vi "readFilterData.vi"() -> ()   [LabVIEW 2026]
uses:
  <vilib>/Utility/miscctls.llb/LVRectTypeDef.ctl
  <vilib>/Utility/miscctls.llb/LVPointTypeDef.ctl
  <userlib>/Sensor.ctl
  <vilib>/Instr/_visa.llb/VISA Configure Serial Port (Instr).vi
panel:
  out "Result 2":dbl
  out "SyncStop 2":bool
  out "Freq Show 2":enum16{"1", "10", "100", "1000"}(ring)
  out "Result":dbl
  in  "UvodniStranka":bool
  in  "ExitApp":bool
  in  "error in (no error)":errorcluster
  in  "Tab Control":T1(tab)
  in  "Playground":bool
  in  "UlohaACC":bool
  in  "UlohaEDA":bool
  in  "UlohaEEG":bool
  in  "UlohaEMG":bool
  in  "UlohaEKG":bool
  out "GraphEKG":waveform(dbl)(graph)
  out "ChartEKG":dbl(graph)
  in  "Vstupní COM port 2":refnum<visa-resource-name>
  in  "Vzorkovací frekvence 2":enum16{"1", "10", "100", "1000"}(ring)
  out "Waveform Graph":waveform(dbl)(graph)
  in  "Cluster":T2
  in  "SendToFilter":bool
  out "Waveform Chart":dbl(graph)
  out "Waveform":waveform(dbl)(graph)
  out "SyncStop":bool
  in  "Vstupní COM port":refnum<visa-resource-name>
  in  "Vzorkovací frekvence (Hz)":enum16{"1", "10", "100", "1000"}(ring)
  in  "Druh signálu":T3
  in  "StartMeasure":bool
  in  "StopMeasure":bool
  in  "Radio Buttons":T4(radio)
  # "Aplikace pro mìøení na platformì PLUX BITalino"
  # "EKG"
  # "EEG"
  # "EDA"
  # "ACC"
  # "EMG"
  # "A1"
  # "A2"
  # "A3"
  # "A4"
  # "A5"
  # "A6"
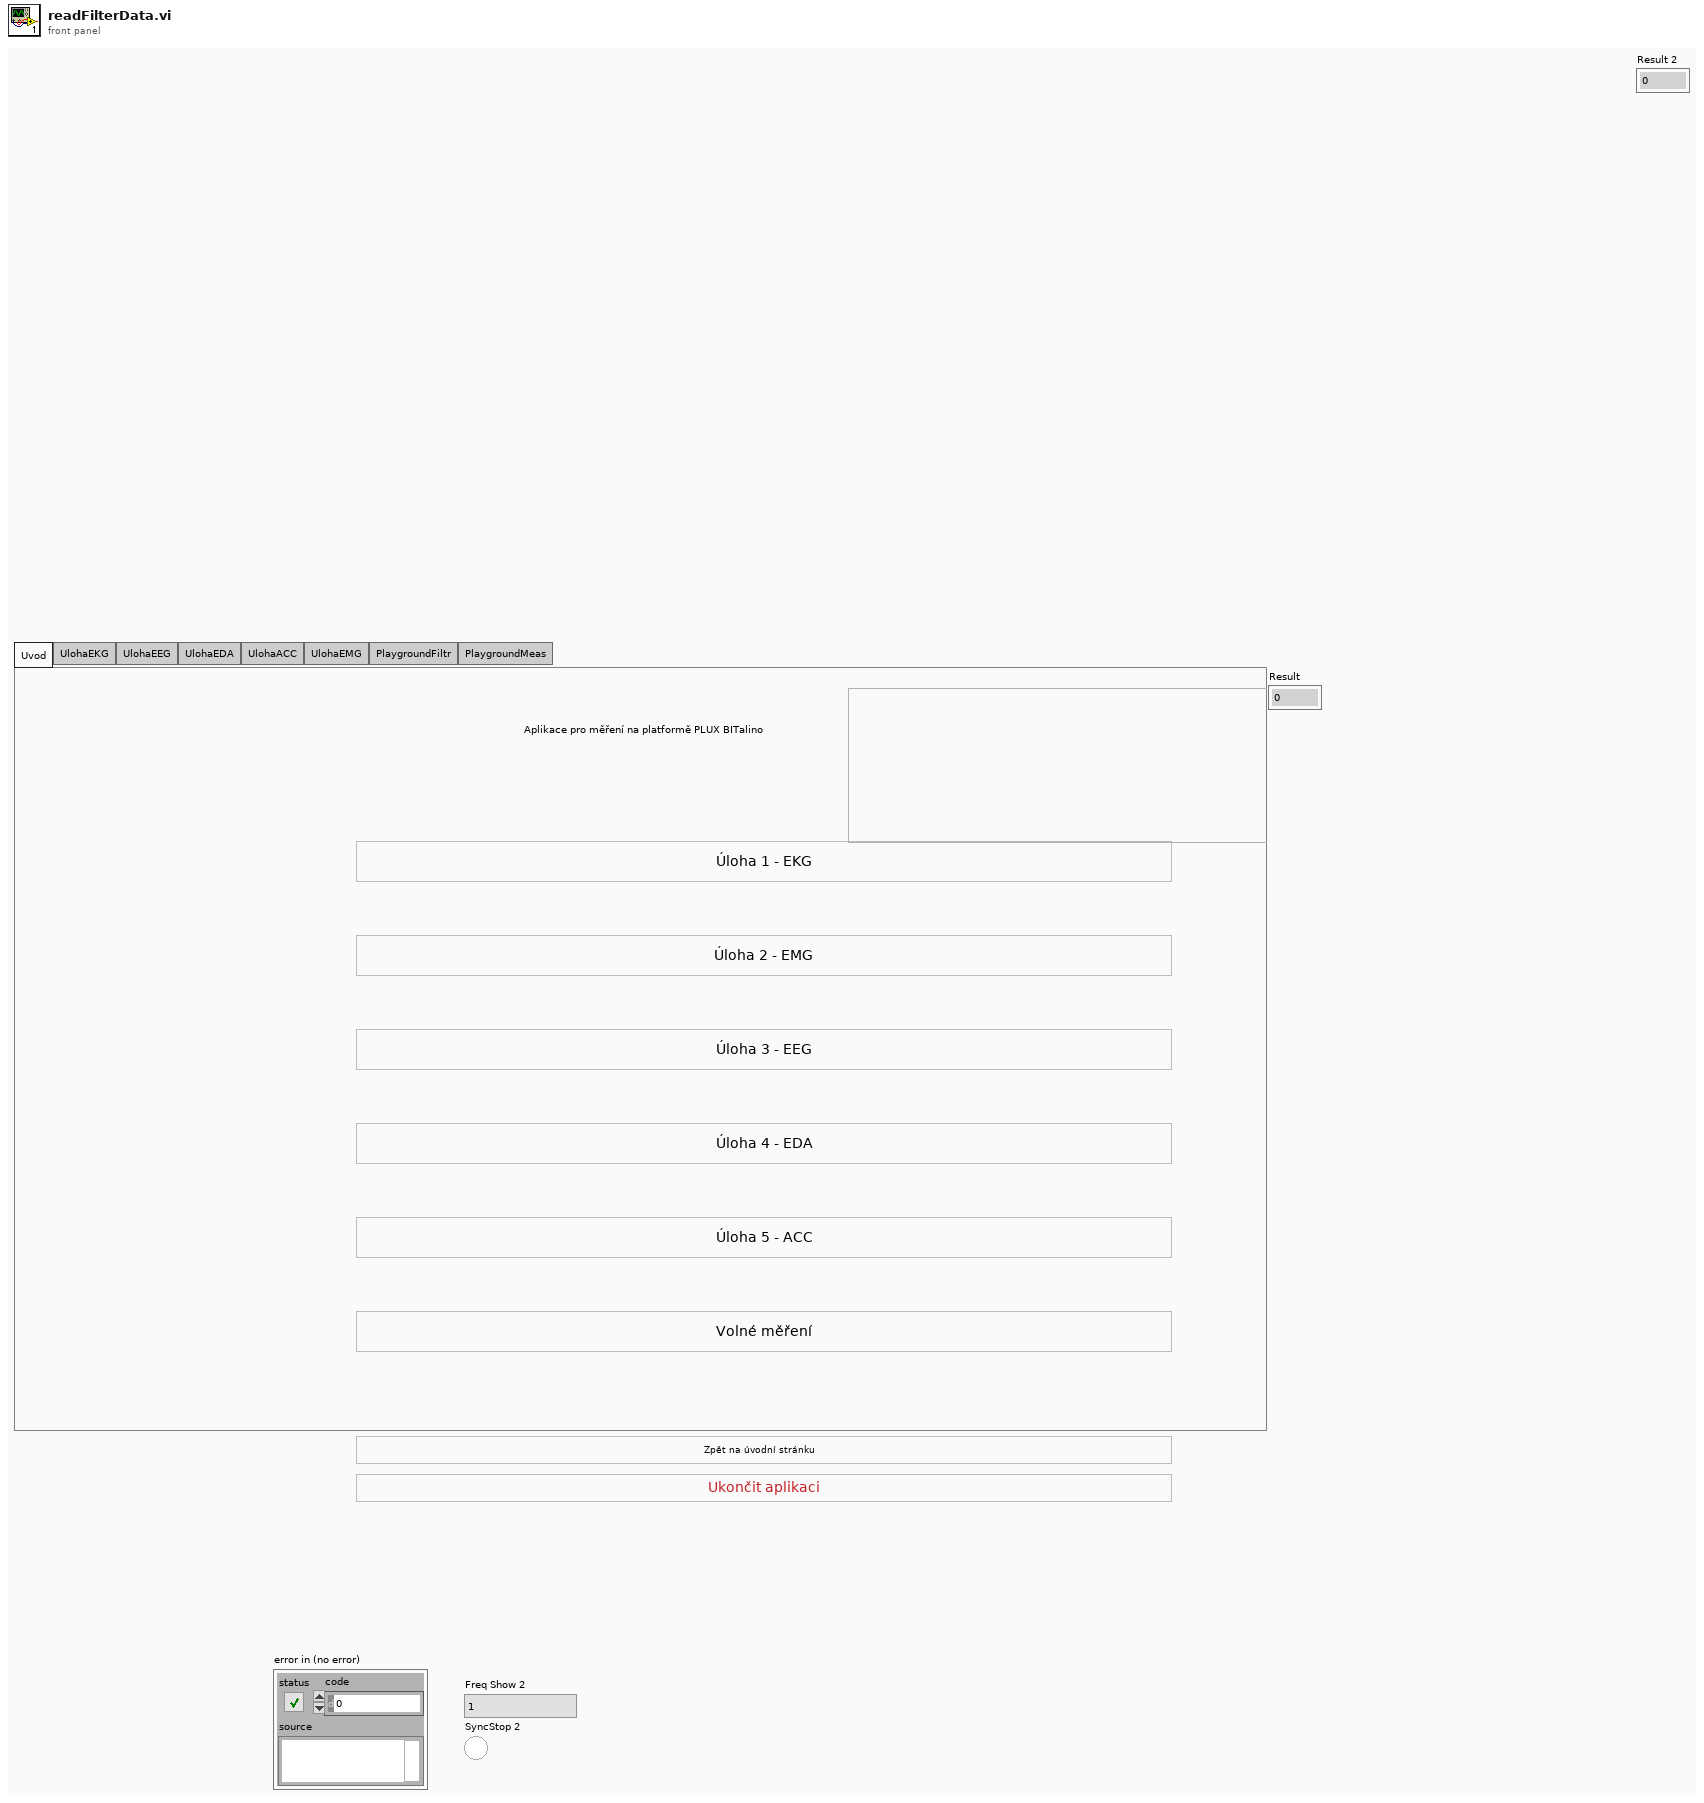
[diagram p1: front panel]
types:
  T1 = enum32{"Uvod", "UlohaEKG", "UlohaEEG", "UlohaEDA", "UlohaACC", "UlohaEMG", "PlaygroundFiltr", "PlaygroundMeas"}
  T2 = cluster{"Horní mezní frekvence":dbl, "Dolní mezní frekvence":dbl, "Filtr":bool, "OdstranitFiltr":bool, "filter type":enum32{"Lowpass", "Highpass", "Bandpass", "Bandstop"}}
  T3 = cluster{"Signál na kanálu A1":enum16{"EMG", "ECG", "EEG", "EDA", "ACC"}, "Signál na kanálu A2":enum16{"EMG", "ECG", "EEG", "EDA", "ACC"}, "Signál na kanálu A3":enum16{"EMG", "ECG", "EEG", "EDA", "ACC"}, "Signál na kanálu A4":enum16{"EMG", "ECG", "EEG", "EDA", "ACC"}, "Signál na kanálu A5":enum16{"EMG", "ECG", "EEG", "EDA", "ACC"}, "Signál na kanálu A6":enum16{"EMG", "ECG", "EEG", "EDA", "ACC"}}
  T4 = enum32{"Item 0", "Item 1", "Item 2", "Item 3", "Item 4", "Item 5"}
  T5 = enum16{"Wait", "Exit", "Measure", "Intro", "UlohaEKG", "UlohaEMG", "PlaygroundMeas", "UlohaEEG", "UlohaEDA", "UlohaACC", "PlaygroundFiltr"}
  T6 = enum16{"Always On", "Always Off", "Off While Running"}
  T7 = enum32{"Uvod", "UlohaEKG", "UlohaEEG", "UlohaEDA", "UlohaACC", "UlohaEMG", "PlaygroundFiltr"}
  T8 = typedef "LVPointTypeDef.ctl" = cluster{"Horizontal":i16, "Vertical":i16}
  T9 = typedef "LVRectTypeDef.ctl" = cluster{"Left":i16, "Top":i16, "Right":i16, "Bottom":i16}
  T10 = enum16{"Wait", "Exit", "Measure", "Intro", "UlohaEKG", "UlohaEMG", "PlaygroundMeas", "UlohaEEG", "UlohaEDA", "UlohaACC"}
  T11 = enum16{"Wait", "Exit", "Measure", "Intro", "UlohaEKG", "UlohaEMG", "PlaygroundMeas"}
  T12 = enum16{"Wait", "Exit", "Measure", "Intro", "UlohaEKG", "UlohaEMG"}
  T13 = enum8{"Enabled", "Disabled", "Disabled and Grayed Out"}
  T14 = typedef "Sensor.ctl" = enum16{"EMG", "ECG", "EEG", "EDA", "ACC", "LUX"}
  T15 = cluster{"Sensor 1":T14, "Sensor 2":T14, "Sensor 3":T14, "Sensor 4":T14, "Sensor 5":T14, "Sensor 6":T14}
  T16 = cluster{"Result":dbl, "Result":dbl, "Result":dbl, "Result":dbl, "Result":dbl, "Result":dbl}
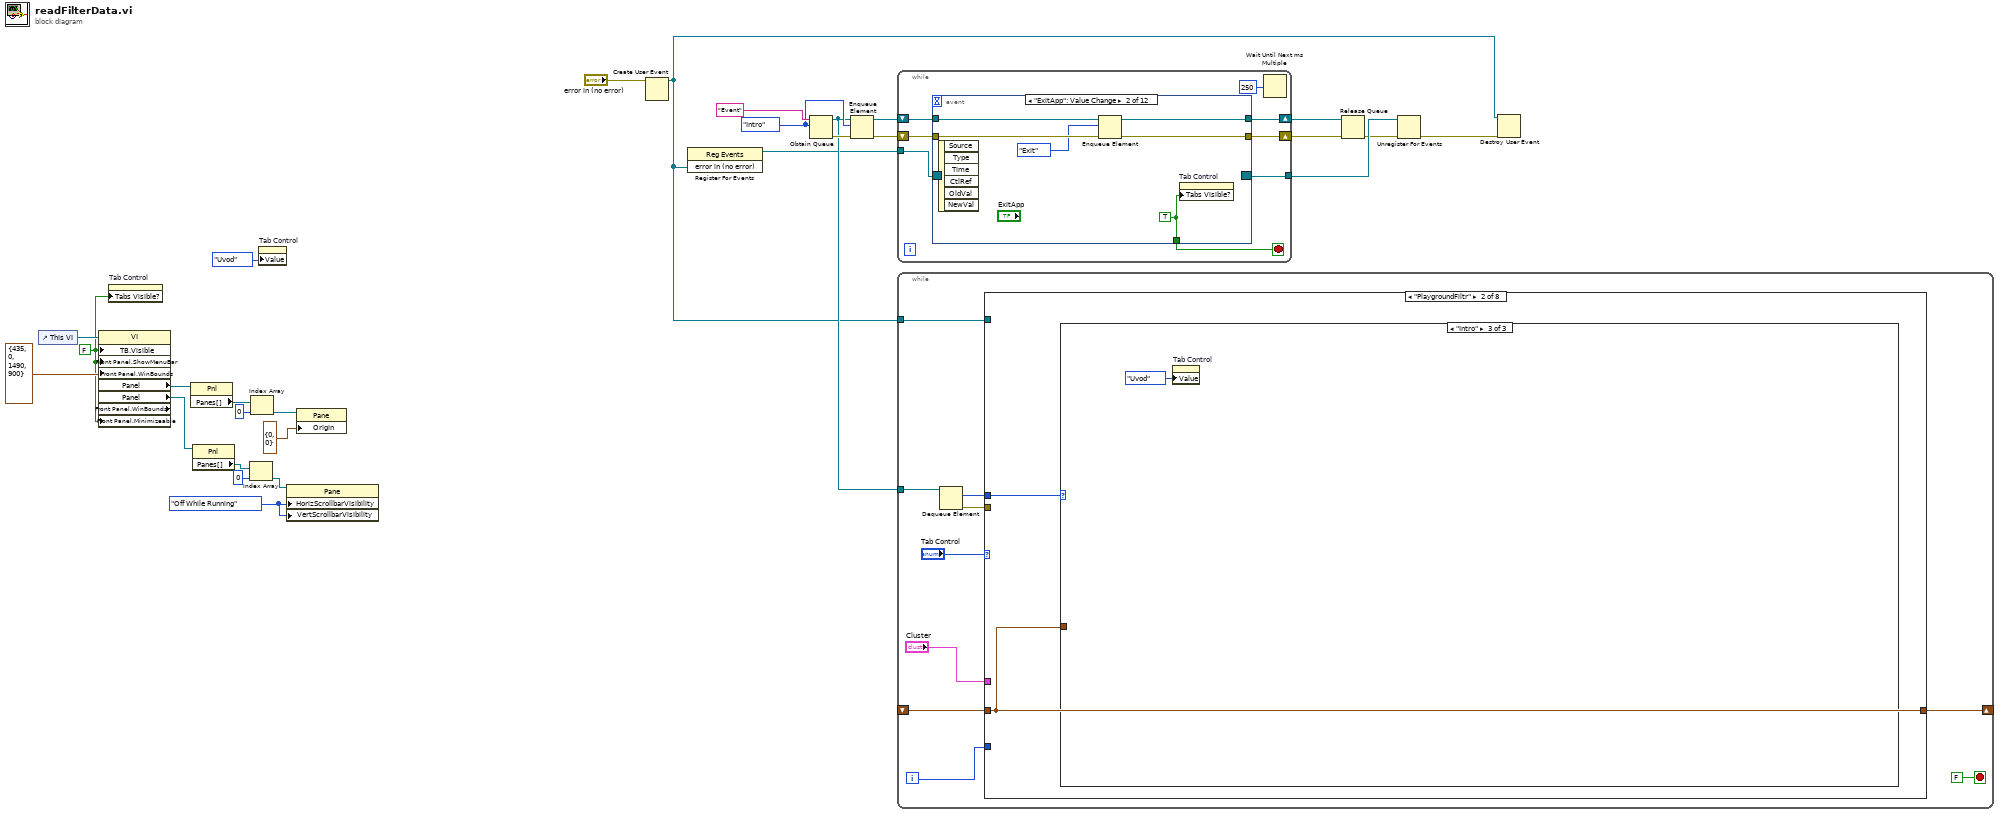
[diagram p0: block diagram]
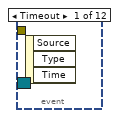
[diagram p2: hidden frame]
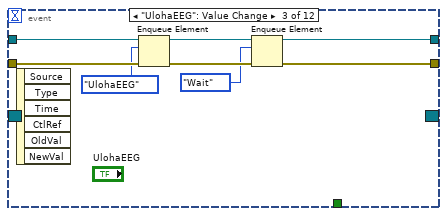
[diagram p3: hidden frame]
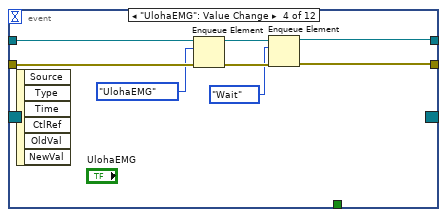
[diagram p4: hidden frame]
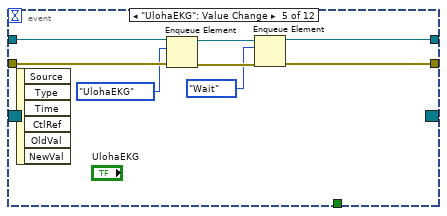
[diagram p5: hidden frame]
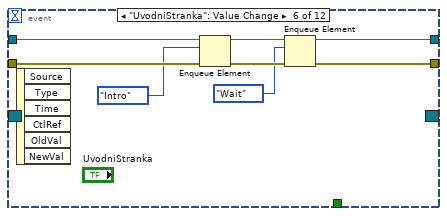
[diagram p6: hidden frame]
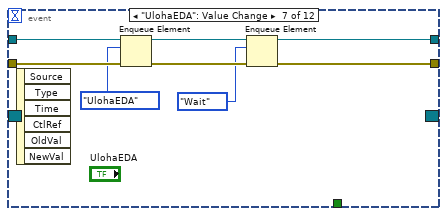
[diagram p7: hidden frame]
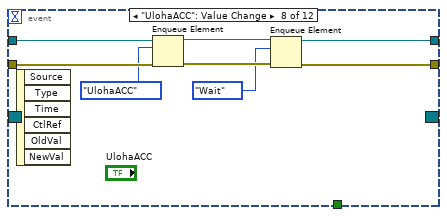
[diagram p8: hidden frame]
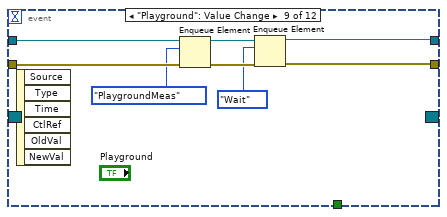
[diagram p9: hidden frame]
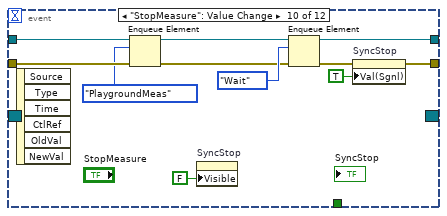
[diagram p10: hidden frame]
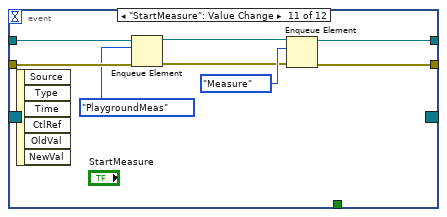
[diagram p11: hidden frame]
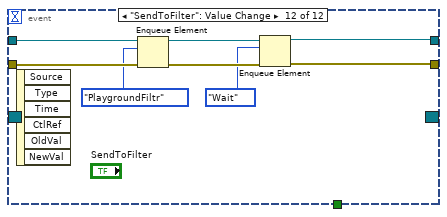
[diagram p12: hidden frame]
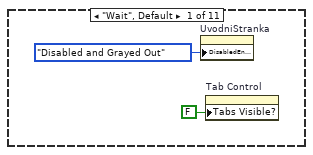
[diagram p14: hidden frame]
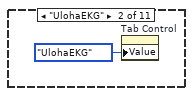
[diagram p15: hidden frame]
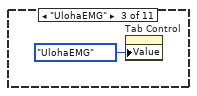
[diagram p16: hidden frame]
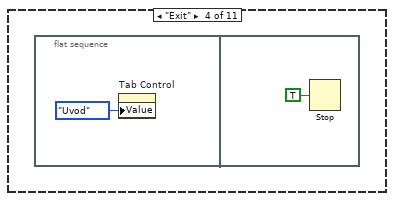
[diagram p17: hidden frame]
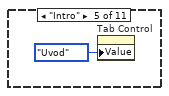
[diagram p18: hidden frame]
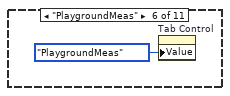
[diagram p19: hidden frame]
diagram:
  w10 = T5."Intro"
  w16 = T6."Off While Running" ("Horizontal Scrollbar Visibility")
  w15 = FALSE ("Front Panel Window:Closeable")
  n1 = control-ref of="This VI"() -> (w28:refnum<vi>)
  n2 = property class="VI" props=["TB.Visible", "Front Panel.ShowMenuBar", "Front Panel.WinBounds", "Panel", "Panel", "Front Panel.WinBounds", "Front Panel.Minimizeable"](reference=w28, "TB.Visible"=w15, "Front Panel.ShowMenuBar"=w15, "Front Panel.WinBounds"=T9 {"Left"=435, "Top"=0, "Right"=1490, "Bottom"=900} ("Front Panel Window:Window Bounds"), "Front Panel.Minimizeable"=w15) -> ("Panel"=w26:refnum<vi>, "Panel"=w20:refnum<vi>)  [unwired: 1 in, 3 out]
  n3 = property on="Tab Control" class="TabCtl (strict)"("Tabs Visible?"=w15) -> ()  [unwired: 2 in, 2 out]
  n4 = property class="Pnl"(reference=w26) -> ("Panes[]"=w25:refnum<vi>[])  [unwired: 1 in, 2 out]
  n5 = property class="Pnl"(reference=w20) -> ("Panes[]"=w19:refnum<vi>[])  [unwired: 1 in, 2 out]
  n6 = Index Array(array=w19, index=0) -> (element=w17:refnum<vi>)
  n7 = Index Array(array=w25, index=0) -> (element=w23:refnum<vi>)
  n8 = property on="Tab Control" class="TabCtl (strict)"("Value"=T7."Uvod" ("Tab Control")) -> ()  [unwired: 2 in, 2 out]
  n9 = property class="Pane"(reference=w17, "HorizScrollbarVisibility"=w16, "VertScrollbarVisibility"=w16) -> ()  [unwired: 1 in, 2 out]
  n10 = property class="Pane"(reference=w23, "Origin"=T8 {"Horizontal"=0, "Vertical"=0}) -> ()  [unwired: 1 in, 2 out]
  n11 = Create User Event(user event datatype="error in (no error)") -> (user event=w2:refnum<user-event>)  [unwired: 1 in, 1 out]
  n12 = register-events(w2) -> (reference out=w1:refnum<event-registration>)  [unwired: 2 in, 1 out]
  n13 = Obtain Queue(name (unnamed)="Event", element data type=w10) -> (queue out=w9:refnum<queue>, error out=w13:errorcluster)  [unwired: 3 in, 1 out]
  n14 = Enqueue Element(queue=w9, element=w10, error in (no error)=w13) -> (queue out=w12:refnum<queue>, error out=w11:errorcluster)  [unwired: 1 in, 1 out]
  n15 = while {
    shift-right: [w34] -> w7
    shift-left: w11 -> [w33]
    shift-right: [w35] -> w8
    shift-left: w12 -> [w36]
    tunnel: [w30] -> w5
    tunnel: w1 -> [w29]
    stop <- w32 stop-if-true
    n16 = event shown="[1] \"ExitApp\": Value Change" {
      selector: w29 -> [_ _ _ _ _ _ _ _ _ _ _ _]
      dyn-events: [_ _ _ _ _ _ _ _ _ _ _ _] -> w30
      timeout: _ -> [_ _ _ _ _ _ _ _ _ _ _ _]
      tunnel: w36 -> [_ w42 w50 w58 w66 w74 w82 w90 w98 w103 w114 w125]
      tunnel: w33 -> [_ w41 w49 w57 w65 w73 w81 w89 w97 w101 w112 w124]
      tunnel: [_ w40 w46 w54 w62 w69 w79 w87 w92 w108 w117 w121] -> w35
      tunnel: [_ w39 w44 w53 w60 w68 w78 w85 w94 w105 w116 w119] -> w34
      tunnel: [_ w37 _ _ _ _ _ _ _ _ _ _] -> w32
      event Timeout {
        n17 = event-data() -> ()  [unwired: 1 in, 3 out]
      }
      event "ExitApp": Value Change {
        w37 = TRUE
        n18 = event-data() -> ()  [unwired: 1 in, 6 out]
        n19 = Enqueue Element(queue=w42, element=enum16{"Wait", "Exit", "Measure"}."Exit", error in (no error)=w41) -> (queue out=w40:refnum<queue>, error out=w39:errorcluster)  [unwired: 1 in, 1 out]
        n20 = property on="Tab Control" class="TabCtl (strict)"("Tabs Visible?"=w37) -> ()  [unwired: 2 in, 2 out]
      }
      event "UlohaEEG": Value Change {
        n21 = event-data() -> ()  [unwired: 1 in, 6 out]
        n22 = Enqueue Element(queue=w50, element=T10."UlohaEEG", error in (no error)=w49) -> (queue out=w47:refnum<queue>, error out=w45:errorcluster)  [unwired: 1 in, 1 out]
        n23 = Enqueue Element(queue=w47, element=T10."Wait", error in (no error)=w45) -> (queue out=w46:refnum<queue>, error out=w44:errorcluster)  [unwired: 1 in, 1 out]
      }
      event "UlohaEMG": Value Change {
        n24 = event-data() -> ()  [unwired: 1 in, 6 out]
        n25 = Enqueue Element(queue=w58, element=T11."UlohaEMG", error in (no error)=w57) -> (queue out=w55:refnum<queue>, error out=w52:errorcluster)  [unwired: 1 in, 1 out]
        n26 = Enqueue Element(queue=w55, element=T11."Wait", error in (no error)=w52) -> (queue out=w54:refnum<queue>, error out=w53:errorcluster)  [unwired: 1 in, 1 out]
      }
      event "UlohaEKG": Value Change {
        n27 = event-data() -> ()  [unwired: 1 in, 6 out]
        n28 = Enqueue Element(queue=w66, element=T12."UlohaEKG", error in (no error)=w65) -> (queue out=w63:refnum<queue>, error out=w61:errorcluster)  [unwired: 1 in, 1 out]
        n29 = Enqueue Element(queue=w63, element=T12."Wait", error in (no error)=w61) -> (queue out=w62:refnum<queue>, error out=w60:errorcluster)  [unwired: 1 in, 1 out]
      }
      event "UvodniStranka": Value Change {
        n30 = event-data() -> ()  [unwired: 1 in, 6 out]
        n31 = Enqueue Element(queue=w74, element=T12."Intro", error in (no error)=w73) -> (queue out=w71:refnum<queue>, error out=w70:errorcluster)  [unwired: 1 in, 1 out]
        n32 = Enqueue Element(queue=w71, element=T12."Wait", error in (no error)=w70) -> (queue out=w69:refnum<queue>, error out=w68:errorcluster)  [unwired: 1 in, 1 out]
      }
      event "UlohaEDA": Value Change {
        n33 = event-data() -> ()  [unwired: 1 in, 6 out]
        n34 = Enqueue Element(queue=w82, element=T10."UlohaEDA", error in (no error)=w81) -> (queue out=w80:refnum<queue>, error out=w77:errorcluster)  [unwired: 1 in, 1 out]
        n35 = Enqueue Element(queue=w80, element=T10."Wait", error in (no error)=w77) -> (queue out=w79:refnum<queue>, error out=w78:errorcluster)  [unwired: 1 in, 1 out]
      }
      event "UlohaACC": Value Change {
        n36 = event-data() -> ()  [unwired: 1 in, 6 out]
        n37 = Enqueue Element(queue=w90, element=T10."UlohaACC", error in (no error)=w89) -> (queue out=w88:refnum<queue>, error out=w86:errorcluster)  [unwired: 1 in, 1 out]
        n38 = Enqueue Element(queue=w88, element=T10."Wait", error in (no error)=w86) -> (queue out=w87:refnum<queue>, error out=w85:errorcluster)  [unwired: 1 in, 1 out]
      }
      event "Playground": Value Change {
        n39 = event-data() -> ()  [unwired: 1 in, 6 out]
        n40 = Enqueue Element(queue=w98, element=T11."PlaygroundMeas", error in (no error)=w97) -> (queue out=w93:refnum<queue>, error out=w95:errorcluster)  [unwired: 1 in, 1 out]
        n41 = Enqueue Element(queue=w93, element=T11."Wait", error in (no error)=w95) -> (queue out=w92:refnum<queue>, error out=w94:errorcluster)  [unwired: 1 in, 1 out]
      }
      event "StopMeasure": Value Change {
        n42 = event-data() -> ()  [unwired: 1 in, 6 out]
        n43 = Enqueue Element(queue=w103, element=T11."PlaygroundMeas", error in (no error)=w101) -> (queue out=w102:refnum<queue>, error out=w100:errorcluster)  [unwired: 1 in, 1 out]
        n44 = property on="SyncStop" class="Bool (strict)"("Visible"=FALSE) -> ()  [unwired: 2 in, 2 out]
        n45 = Enqueue Element(queue=w102, element=enum16{"Wait", "Exit", "Measure"}."Wait", error in (no error)=w100) -> (queue out=w108:refnum<queue>, error out=w106:errorcluster)  [unwired: 1 in, 1 out]
        n46 = property on="SyncStop" class="Bool (strict)"(error in=w106, "Val(Sgnl)"=TRUE ("Value (Signaling)")) -> (error out=w105:errorcluster)  [unwired: 1 in, 1 out]
      }
      event "StartMeasure": Value Change {
        n47 = event-data() -> ()  [unwired: 1 in, 6 out]
        n48 = Enqueue Element(queue=w114, element=T11."PlaygroundMeas", error in (no error)=w112) -> (queue out=w113:refnum<queue>, error out=w111:errorcluster)  [unwired: 1 in, 1 out]
        n49 = Enqueue Element(queue=w113, element=enum16{"Wait", "Exit", "Measure"}."Measure", error in (no error)=w111) -> (queue out=w117:refnum<queue>, error out=w116:errorcluster)  [unwired: 1 in, 1 out]
      }
      event "SendToFilter": Value Change {
        n50 = event-data() -> ()  [unwired: 1 in, 6 out]
        n51 = Enqueue Element(queue=w125, element=T5."PlaygroundFiltr", error in (no error)=w124) -> (queue out=w122:refnum<queue>, error out=w120:errorcluster)  [unwired: 1 in, 1 out]
        n52 = Enqueue Element(queue=w122, element=T5."Wait", error in (no error)=w120) -> (queue out=w121:refnum<queue>, error out=w119:errorcluster)  [unwired: 1 in, 1 out]
      }
    }
    n53 = Wait Until Next ms Multiple(millisecond multiple=u32 250) -> ()  [unwired: 1 out]
  }
  n54 = while {
    shift-right: [w135] -> _
    shift-left: _ -> [w134]
    tunnel: w9 -> [w129]
    tunnel: w2 -> [w128]
    i -> [w132]
    stop <- FALSE stop-if-true
    n55 = Dequeue Element(queue=w129) -> (element=w130:T5, error out=w127:errorcluster)  [unwired: 2 in, 2 out]
    n56 = case shown="\"PlaygroundFiltr\"" "Tab Control" {
      tunnel: [w137 w149 w158 w223 w229 w235 w241 w247] -> w135
      tunnel: w134 -> [w137 w149 w158 w223 w229 w235 w241 w246]
      tunnel: "Cluster" -> [_ _ _ _ _ _ _ _]
      tunnel: w132 -> [_ _ _ _ _ _ _ _]
      tunnel: w130 -> [w136 w150 w157 w222 w228 w234 w240 w250]
      tunnel: w128 -> [_ _ w156 _ _ _ _ w249]
      tunnel: w127 -> [_ _ _ _ _ _ _ w248]
      frame "Uvod", Default {
        n57 = case shown="\"PlaygroundFiltr\"" w136 {
          frame "Wait", Default {
            n58 = property on="UvodniStranka" class="Bool"("DisabledEnum"=T13."Disabled and Grayed Out" ("Disabled")) -> ()  [unwired: 2 in, 2 out]
            n59 = property on="Tab Control" class="TabCtl (strict)"("Tabs Visible?"=FALSE) -> ()  [unwired: 2 in, 2 out]
          }
          frame "UlohaEKG" {
            n60 = property on="Tab Control" class="TabCtl (strict)"("Value"=T1."UlohaEKG" ("Tab Control")) -> ()  [unwired: 2 in, 2 out]
          }
          frame "UlohaEMG" {
            n61 = property on="Tab Control" class="TabCtl (strict)"("Value"=T1."UlohaEMG" ("Tab Control")) -> ()  [unwired: 2 in, 2 out]
          }
          frame "Exit" {
            n62 = flat-sequence {
              frame #0 {
                n63 = property on="Tab Control" class="TabCtl (strict)"("Value"=T1."Uvod" ("Tab Control")) -> ()  [unwired: 2 in, 2 out]
              }
              frame #1 {
                n64 = Stop(stop? (T)=TRUE) -> ()
              }
            }
          }
          frame "Intro" {
            n65 = property on="Tab Control" class="TabCtl (strict)"("Value"=T1."Uvod" ("Tab Control")) -> ()  [unwired: 2 in, 2 out]
          }
          frame "PlaygroundMeas" {
            n66 = property on="Tab Control" class="TabCtl (strict)"("Value"=T1."PlaygroundMeas" ("Tab Control")) -> ()  [unwired: 2 in, 2 out]
          }
          frame "Measure" {
          }
          frame "UlohaEEG" {
            n67 = property on="Tab Control" class="TabCtl (strict)"("Value"=T1."UlohaEEG" ("Tab Control")) -> ()  [unwired: 2 in, 2 out]
          }
          frame "UlohaEDA" {
            n68 = property on="Tab Control" class="TabCtl (strict)"("Value"=T1."UlohaEDA" ("Tab Control")) -> ()  [unwired: 2 in, 2 out]
          }
          frame "UlohaACC" {
            n69 = property on="Tab Control" class="TabCtl (strict)"("Value"=T1."UlohaACC" ("Tab Control")) -> ()  [unwired: 2 in, 2 out]
          }
          frame "PlaygroundFiltr" {
          }
        }
      }
      frame "PlaygroundFiltr" {
        n70 = case shown="\"Intro\"" w150 {
          tunnel: w149 -> [w151 _ _]
          frame "Wait", Default {
            n71 = property on="UvodniStranka" class="Bool"("DisabledEnum"=T13."Enabled" ("Disabled")) -> ()  [unwired: 2 in, 2 out]
            "Waveform Graph" <- w151
          }
          frame "Exit" {
            n72 = flat-sequence {
              frame #0 {
                n73 = property on="Tab Control" class="TabCtl (strict)"("Value"=T1."Uvod" ("Tab Control")) -> ()  [unwired: 2 in, 2 out]
              }
              frame #1 {
                n74 = Stop(stop? (T)=TRUE) -> ()
              }
            }
          }
          frame "Intro" {
            n75 = property on="Tab Control" class="TabCtl (strict)"("Value"=T1."Uvod" ("Tab Control")) -> ()  [unwired: 2 in, 2 out]
          }
        }
      }
      frame "UlohaEKG" {
        n76 = case shown="\"Intro\"" w157 {
          tunnel: w156 -> [_ _ w166 _ _ _]
          frame "Wait", Default {
            n77 = property on="UvodniStranka" class="Bool"("DisabledEnum"=T13."Enabled" ("Disabled")) -> ()  [unwired: 2 in, 2 out]
          }
          frame "Exit" {
            n78 = flat-sequence {
              frame #0 {
                n79 = property on="Tab Control" class="TabCtl (strict)"("Value"=T1."Uvod" ("Tab Control")) -> ()  [unwired: 2 in, 2 out]
              }
              frame #1 {
                n80 = Stop(stop? (T)=TRUE) -> ()
              }
            }
          }
          frame "Measure" {
            w169 = "Signal" ("name (unnamed)")
            n81 = call-poly "VISA Configure Serial Port"("VISA resource name"="Vstupní COM port 2", "timeout (10sec)"=u32 2000, "baud rate (9600)"=u32 115200) -> ("VISA resource name out"=w186:refnum<visa-resource-name>, "error out"=w185:errorcluster)  [unwired: 11 in]
            n82 = call "InitBITalino.vi"("Battery \nThreshold (%)"=u8 5 ("Battery \nThreshold (%)"), "MODE"=FALSE, "error in (no error)"=w185, "Sample Rate"="Vzorkovací frekvence 2", "BITalino"=w186) -> ("error out"=w181:errorcluster, "VISA out"=w182:refnum<visa-resource-name>)  [unwired: 4 in, 1 out]
            n83 = Obtain Queue(name (unnamed)=w169, element data type=w169, error in (no error)=w181) -> (queue out=w165:refnum<queue>, error out=w180:errorcluster)  [unwired: 2 in, 1 out]
            n84 = while {
              tunnel: w165 -> [w194]
              tunnel: [w190] -> w164 mode=indexing
              stop <- w191 stop-if-true
              n85 = Dequeue Element(queue=w194) -> (element=w193:string, error out=w192:errorcluster)  [unwired: 2 in, 2 out]
              n86 = case shown="No Error" w192 {
                tunnel: w193 -> [w203 _]
                tunnel: [FALSE TRUE] -> w191
                tunnel: [w197 w204] -> w190
                frame No Error {
                  n87 = call "Packet Read.vi"("Packets"=w203) -> ("Analog Channels"=w202:cluster{u16, u16, u16, u16, u16, u16})  [unwired: 7 in, 3 out]
                  n88 = call "Conversion.vi"("Sensor Type"=T15 {"Sensor 1"=enum."ECG", "Sensor 2"=enum."ECG", "Sensor 3"=enum."ECG", "Sensor 4"=enum."ECG", "Sensor 5"=enum."ECG", "Sensor 6"=enum."ECG"}, "Analog Channels"=w202) -> ("output cluster"=w200:T16)  [unwired: 8 in, 1 out]
                  n89 = Cluster To Array(cluster=w200) -> (array=w199:dbl[])
                  n90 = Unbundle(w200) -> ("Result"=w197:dbl)  [unwired: 5 out]
                  "Result 2" <- w197
                  n91 = Index Array(array=w199, index=2) -> (element=→"ChartEKG":dbl)
                }
                frame Error {
                  n92 = local read "Result 2"() -> (w204:dbl)
                }
              }
            }
            n93 = while {
              shift-right: [w214] -> w178
              shift-left: w182 -> [w220]
              shift-right: [w209] -> w179
              shift-left: w180 -> [w219]
              shift-right: [w210] -> w173
              shift-left: w165 -> [w213]
              stop <- w208 stop-if-true
              n94 = VISA Write(VISA resource name=w220, write buffer="0x03", error in (no error)=w219) -> (VISA resource name out=w217:refnum<visa-resource-name>, error out=w216:errorcluster)  [unwired: 1 out]
              n95 = VISA Read(VISA resource name=w217, byte count=u32 8, error in (no error)=w216) -> (VISA resource name out=w214:refnum<visa-resource-name>, read buffer=w212:string, error out=w211:errorcluster)  [unwired: 1 out]
              n96 = Enqueue Element(queue=w213, element=w212, error in (no error)=w211) -> (queue out=w210:refnum<queue>, error out=w209:errorcluster)  [unwired: 1 in, 1 out]
              n97 = local read "SyncStop 2"() -> (w206:bool)
              n98 = Unbundle By Name(w209) -> ("status"=w207:bool)
              n99 = Or(x=w207, y=w206) -> (x .or. y?=w208:bool)
            }
            n100 = call "Wait.vi"("error in (no error)"=w179) -> ("error out"=w175:errorcluster)  [unwired: 10 in]
            n101 = Build Array(u8 0) -> (w171:u8[])
            n102 = Byte Array To String(unsigned byte array=w171) -> (string=w170:string)
            n103 = VISA Write(VISA resource name=w178, write buffer=w170, error in (no error)=w175) -> (VISA resource name out=w177:refnum<visa-resource-name>, error out=w176:errorcluster)  [unwired: 1 out]
            n104 = VISA Close(VISA resource name=w177, error in (no error)=w176) -> (error out=w174:errorcluster)
            n105 = Bundle By Name("Y"=w164, "dt"=0.001) -> (→"GraphEKG":waveform(dbl))  [unwired: 1 in]
            n106 = Release Queue(queue=w173, error in (no error)=w174) -> (error out=w168:errorcluster)  [unwired: 1 in, 2 out]
            n107 = Generate User Event(user event=w166, event data cluster=w168) -> ()  [unwired: 2 in, 2 out]
            "Freq Show 2" <- "Vzorkovací frekvence 2"
          }
          frame "Intro" {
            n108 = property on="Tab Control" class="TabCtl (strict)"("Value"=T1."Uvod" ("Tab Control")) -> ()  [unwired: 2 in, 2 out]
          }
          frame "UlohaEKG" {
          }
          frame "UlohaEMG" {
          }
        }
      }
      frame "UlohaEEG" {
        n109 = case shown="\"Exit\"" w222 {
          frame "Wait", Default {
            n110 = property on="UvodniStranka" class="Bool"("DisabledEnum"=T13."Enabled" ("Disabled")) -> ()  [unwired: 2 in, 2 out]
          }
          frame "Exit" {
            n111 = flat-sequence {
              frame #0 {
                n112 = property on="Tab Control" class="TabCtl (strict)"("Value"=T1."Uvod" ("Tab Control")) -> ()  [unwired: 2 in, 2 out]
              }
              frame #1 {
                n113 = Stop(stop? (T)=TRUE) -> ()
              }
            }
          }
          frame "Measure" {
          }
          frame "Intro" {
            n114 = property on="Tab Control" class="TabCtl (strict)"("Value"=T1."Uvod" ("Tab Control")) -> ()  [unwired: 2 in, 2 out]
          }
          frame "UlohaEKG" {
          }
          frame "UlohaEMG" {
          }
          frame "PlaygroundMeas" {
          }
          frame "UlohaEEG" {
          }
          frame "UlohaEDA" {
          }
          frame "UlohaACC" {
          }
        }
      }
      frame "UlohaEDA" {
        n115 = case shown="\"Wait\", Default" w228 {
          frame "Wait", Default {
            n116 = property on="UvodniStranka" class="Bool"("DisabledEnum"=T13."Enabled" ("Disabled")) -> ()  [unwired: 2 in, 2 out]
          }
          frame "Exit" {
            n117 = flat-sequence {
              frame #0 {
                n118 = property on="Tab Control" class="TabCtl (strict)"("Value"=T1."Uvod" ("Tab Control")) -> ()  [unwired: 2 in, 2 out]
              }
              frame #1 {
                n119 = Stop(stop? (T)=TRUE) -> ()
              }
            }
          }
          frame "Measure" {
          }
          frame "Intro" {
            n120 = property on="Tab Control" class="TabCtl (strict)"("Value"=T1."Uvod" ("Tab Control")) -> ()  [unwired: 2 in, 2 out]
          }
          frame "UlohaEKG" {
          }
          frame "UlohaEMG" {
          }
          frame "PlaygroundMeas" {
          }
          frame "UlohaEEG" {
          }
          frame "UlohaEDA" {
          }
          frame "UlohaACC" {
          }
        }
      }
      frame "UlohaACC" {
        n121 = case shown="\"Wait\", Default" w234 {
          frame "Wait", Default {
            n122 = property on="UvodniStranka" class="Bool"("DisabledEnum"=T13."Enabled" ("Disabled")) -> ()  [unwired: 2 in, 2 out]
          }
          frame "Exit" {
            n123 = flat-sequence {
              frame #0 {
                n124 = property on="Tab Control" class="TabCtl (strict)"("Value"=T1."Uvod" ("Tab Control")) -> ()  [unwired: 2 in, 2 out]
              }
              frame #1 {
                n125 = Stop(stop? (T)=TRUE) -> ()
              }
            }
          }
          frame "Measure" {
          }
          frame "Intro" {
            n126 = property on="Tab Control" class="TabCtl (strict)"("Value"=T1."Uvod" ("Tab Control")) -> ()  [unwired: 2 in, 2 out]
          }
          frame "UlohaEKG" {
          }
          frame "UlohaEMG" {
          }
          frame "PlaygroundMeas" {
          }
          frame "UlohaEEG" {
          }
          frame "UlohaEDA" {
          }
          frame "UlohaACC" {
          }
        }
      }
      frame "UlohaEMG" {
        n127 = case shown="\"Intro\"" w240 {
          frame "Wait", Default {
            n128 = property on="UvodniStranka" class="Bool"("DisabledEnum"=T13."Enabled" ("Disabled")) -> ()  [unwired: 2 in, 2 out]
          }
          frame "Exit" {
            n129 = flat-sequence {
              frame #0 {
                n130 = property on="Tab Control" class="TabCtl (strict)"("Value"=T1."Uvod" ("Tab Control")) -> ()  [unwired: 2 in, 2 out]
              }
              frame #1 {
                n131 = Stop(stop? (T)=TRUE) -> ()
              }
            }
          }
          frame "Measure" {
          }
          frame "Intro" {
            n132 = property on="Tab Control" class="TabCtl (strict)"("Value"=T1."Uvod" ("Tab Control")) -> ()  [unwired: 2 in, 2 out]
          }
          frame "UlohaEKG" {
          }
          frame "UlohaEMG" {
          }
          frame "PlaygroundMeas" {
          }
        }
      }
      frame "PlaygroundMeas" {
        n133 = case shown="No Error" w248 {
          tunnel: w250 -> [w255 _]
          tunnel: [FALSE TRUE] -> _
          tunnel: w249 -> [w253 _]
          tunnel: [w252 w363] -> w247
          tunnel: w246 -> [w251 w363]
          frame No Error {
            n134 = case shown="\"PlaygroundFiltr\"" w255 {
              tunnel: w253 -> [_ _ _ _ w273]
              tunnel: [w256 w259 w262 w264 w267] -> w252
              tunnel: w251 -> [w256 w259 w262 w264 _]
              frame "Wait", Default {
                n135 = property on="UvodniStranka" class="Bool"("DisabledEnum"=T13."Enabled" ("Disabled")) -> ()  [unwired: 2 in, 2 out]
                n136 = property on="SyncStop" class="Bool (strict)"("Val(Sgnl)"=FALSE ("Value (Signaling)")) -> ()  [unwired: 2 in, 2 out]
              }
              frame "Exit" {
                n137 = flat-sequence {
                  frame #0 {
                    n138 = property on="Tab Control" class="TabCtl (strict)"("Value"=T1."Uvod" ("Tab Control")) -> ()  [unwired: 2 in, 2 out]
                  }
                  frame #1 {
                    n139 = Stop(stop? (T)=TRUE) -> ()
                  }
                }
              }
              frame "PlaygroundFiltr" {
                n140 = property on="Tab Control" class="TabCtl (strict)"("Value"=T1."PlaygroundFiltr" ("Tab Control")) -> ()  [unwired: 2 in, 2 out]
              }
              frame "Intro" {
                n141 = flat-sequence {
                  frame #0 {
                    n142 = property on="Tab Control" class="TabCtl (strict)"("Value"=T1."Uvod" ("Tab Control")) -> ()  [unwired: 2 in, 2 out]
                  }
                  frame #1 {
                    n143 = Wait (ms)(milliseconds to wait=u32 100) -> ()  [unwired: 1 out]
                  }
                }
              }
              frame "Measure" {
                w275 = "Signal" ("name (unnamed)")
                n144 = Reciprocal(x="Vzorkovací frekvence (Hz)") -> (1/x=w268:dbl)
                n145 = call-poly "VISA Configure Serial Port"("VISA resource name"="Vstupní COM port", "timeout (10sec)"=u32 2000, "baud rate (9600)"=u32 115200) -> ("VISA resource name out"=w292:refnum<visa-resource-name>, "error out"=w291:errorcluster)  [unwired: 11 in]
                n146 = property on="Waveform Chart" class="WFChart (strict)"("XScale.Multiplier"=w268) -> ()  [unwired: 2 in, 2 out]
                n147 = call "InitBITalino.vi"("Battery \nThreshold (%)"=u8 5 ("Battery \nThreshold (%)"), "MODE"=FALSE, "error in (no error)"=w291, "Sample Rate"="Vzorkovací frekvence (Hz)", "BITalino"=w292) -> ("error out"=w287:errorcluster, "VISA out"=w288:refnum<visa-resource-name>)  [unwired: 4 in, 1 out]
                n148 = Obtain Queue(name (unnamed)=w275, element data type=w275, error in (no error)=w287) -> (queue out=w274:refnum<queue>, error out=w286:errorcluster)  [unwired: 2 in, 1 out]
                n149 = while {
                  shift-right: [w356] -> w284
                  shift-left: w288 -> [w362]
                  shift-right: [w351] -> w285
                  shift-left: w286 -> [w361]
                  shift-right: [w352] -> w279
                  shift-left: w274 -> [w355]
                  stop <- w350 stop-if-true
                  n150 = VISA Write(VISA resource name=w362, write buffer="0x03", error in (no error)=w361) -> (VISA resource name out=w359:refnum<visa-resource-name>, error out=w358:errorcluster)  [unwired: 1 out]
                  n151 = VISA Read(VISA resource name=w359, byte count=u32 8, error in (no error)=w358) -> (VISA resource name out=w356:refnum<visa-resource-name>, read buffer=w354:string, error out=w353:errorcluster)  [unwired: 1 out]
                  n152 = Enqueue Element(queue=w355, element=w354, error in (no error)=w353) -> (queue out=w352:refnum<queue>, error out=w351:errorcluster)  [unwired: 1 in, 1 out]
                  n153 = local read "SyncStop"() -> (w348:bool)
                  n154 = Unbundle By Name(w351) -> ("status"=w349:bool)
                  n155 = Or(x=w349, y=w348) -> (x .or. y?=w350:bool)
                }
                n156 = while {
                  tunnel: w274 -> [w301]
                  tunnel: [w297] -> w271 mode=indexing
                  tunnel: "Radio Buttons" -> [w296]
                  stop <- w298 stop-if-true
                  n157 = Dequeue Element(queue=w301) -> (element=w300:string, error out=w299:errorcluster)  [unwired: 2 in, 2 out]
                  n158 = case shown="No Error" w299 {
                    tunnel: w300 -> [w308 _]
                    tunnel: [FALSE TRUE] -> w298
                    tunnel: [w303 w346] -> w297
                    tunnel: w296 -> [w305 _]
                    frame No Error {
                      n159 = call "Packet Read.vi"("Packets"=w308) -> ("Analog Channels"=w307:cluster{u16, u16, u16, u16, u16, u16})  [unwired: 7 in, 3 out]
                      n160 = call "Conversion.vi"("Sensor Type"="Druh signálu", "Analog Channels"=w307) -> ("output cluster"=w304:T16)  [unwired: 8 in, 1 out]
                      n161 = case shown="\"Item 0\", Default" w305 {
                        tunnel: w304 -> [w315 w322 w327 w332 w337 w342]
                        tunnel: [w312 w321 w326 w331 w336 w341] -> w303
                        tunnel: "Druh signálu" -> [w310 _ _ _ _ _]
                        frame "Item 0", Default {
                          n162 = Unbundle(w310) -> ("Signál na kanálu A1"=w309:enum16{"EMG", "ECG", "EEG", "EDA", "ACC"})  [unwired: 5 out]
                          n163 = Cluster To Array(cluster=w315) -> (array=w314:dbl[])
                          n164 = case shown="\"EMG\", Default" w309 {
                            frame "EMG", Default {
                              n165 = property on="Waveform Chart" class="WFChart (strict)"("XScale.NameLbl.Text"="amplituda (mV)" ("X Scale.Name Label.Text")) -> ()  [unwired: 2 in, 2 out]
                            }
                            frame "ECG" {
                              n166 = property on="Waveform Chart" class="WFChart (strict)"("XScale.NameLbl.Text"="amplituda (mV)" ("X Scale.Name Label.Text")) -> ()  [unwired: 2 in, 2 out]
                            }
                            frame "EEG" {
                              n167 = property on="Waveform Chart" class="WFChart (strict)"("XScale.NameLbl.Text"="amplituda (uV)" ("X Scale.Name Label.Text")) -> ()  [unwired: 2 in, 2 out]
                            }
                            frame "EDA" {
                              n168 = property on="Waveform Chart" class="WFChart (strict)"("XScale.NameLbl.Text"="amplitude (mS)" ("X Scale.Name Label.Text")) -> ()  [unwired: 2 in, 2 out]
                            }
                            frame "ACC" {
                              n169 = property on="Waveform Chart" class="WFChart (strict)"("XScale.NameLbl.Text"="amplituda (g)" ("X Scale.Name Label.Text")) -> ()  [unwired: 2 in, 2 out]
                            }
                          }
                          n170 = Index Array(array=w314, index=0) -> (element=→"Waveform Chart":dbl)
                          n171 = Unbundle(w315) -> ("Result"=w312:dbl)  [unwired: 5 out]
                        }
                        frame "Item 1" {
                          n172 = Cluster To Array(cluster=w322) -> (array=w325:dbl[])
                          n173 = Index Array(array=w325, index=1) -> (element=w323:dbl)
                          n174 = local write "Waveform Chart"(w323) -> ()
                          n175 = Unbundle(w322) -> ("Result"=w321:dbl)  [unwired: 5 out]
                        }
                        frame "Item 2" {
                          n176 = Cluster To Array(cluster=w327) -> (array=w330:dbl[])
                          n177 = Unbundle(w327) -> ("Result"=w326:dbl)  [unwired: 5 out]
                          n178 = Index Array(array=w330, index=2) -> (element=w328:dbl)
                          n179 = local write "Waveform Chart"(w328) -> ()
                        }
                        frame "Item 3" {
                          n180 = Cluster To Array(cluster=w332) -> (array=w335:dbl[])
                          n181 = Unbundle(w332) -> ("Result"=w331:dbl)  [unwired: 5 out]
                          n182 = Index Array(array=w335, index=3) -> (element=w333:dbl)
                          n183 = local write "Waveform Chart"(w333) -> ()
                        }
                        frame "Item 4" {
                          n184 = Cluster To Array(cluster=w337) -> (array=w340:dbl[])
                          n185 = Unbundle(w337) -> ("Result"=w336:dbl)  [unwired: 5 out]
                          n186 = Index Array(array=w340, index=4) -> (element=w338:dbl)
                          n187 = local write "Waveform Chart"(w338) -> ()
                        }
                        frame "Item 5" {
                          n188 = Cluster To Array(cluster=w342) -> (array=w345:dbl[])
                          n189 = Unbundle(w342) -> ("Result"=w341:dbl)  [unwired: 5 out]
                          n190 = Index Array(array=w345, index=5) -> (element=w343:dbl)
                          n191 = local write "Waveform Chart"(w343) -> ()
                        }
                      }
                      "Result" <- w303
                    }
                    frame Error {
                      n192 = local read "Result"() -> (w346:dbl)
                    }
                  }
                }
                n193 = call "Wait.vi"("error in (no error)"=w285) -> ("error out"=w281:errorcluster)  [unwired: 10 in]
                n194 = Build Array(u8 0) -> (w277:u8[])
                n195 = Byte Array To String(unsigned byte array=w277) -> (string=w276:string)
                n196 = VISA Write(VISA resource name=w284, write buffer=w276, error in (no error)=w281) -> (VISA resource name out=w283:refnum<visa-resource-name>, error out=w282:errorcluster)  [unwired: 1 out]
                n197 = VISA Close(VISA resource name=w283, error in (no error)=w282) -> (error out=w280:errorcluster)
                n198 = Release Queue(queue=w279, error in (no error)=w280) -> (error out=w272:errorcluster)  [unwired: 1 in, 2 out]
                n199 = Generate User Event(user event=w273, event data cluster=w272) -> ()  [unwired: 2 in, 2 out]
                n200 = Bundle By Name("Y"=w271, "dt"=w268) -> (w267:waveform(dbl))  [unwired: 1 in]
                "Waveform" <- w267
              }
            }
          }
          frame Error {
          }
        }
      }
    }
  }
  n201 = Release Queue(queue=w8, error in (no error)=w7) -> (error out=w4:errorcluster)  [unwired: 1 in, 2 out]
  n202 = Unregister For Events(event registration refnum=w5, error in=w4) -> (error out=w3:errorcluster)
  n203 = Destroy User Event(user event=w2, error in=w3) -> ()  [unwired: 1 out]
